vi "saveAllScanScripts.vi"(6 "scanType":string, 8 "error in (no error)":errorcluster, 9 "Values":string[](array[string]), 10 "scriptListArray":refnum<class "ScriptEventList.lvclass">[](array[class]), 11 "ScriptEditorV2 in":refnum<class "ScriptEditorV2.lvclass">) -> (0 "error out":errorcluster, 3 "ScriptEditorV2 out":refnum<class "ScriptEditorV2.lvclass">)   [LabVIEW 2009, in "Views.lvlib" / "ScriptEditor.lvlib" / "ScriptEditorV2.lvclass"]
uses:
  ScriptEditorV2.lvclass
  Tools/Scripting/ScriptingEvent/ScriptEventList/ScriptEventList.lvclass
  ScriptEditorV2.lvclass/ScriptEditorV2.ctl
  Tools/Scripting/DataPointScript/DataPointScript.lvclass
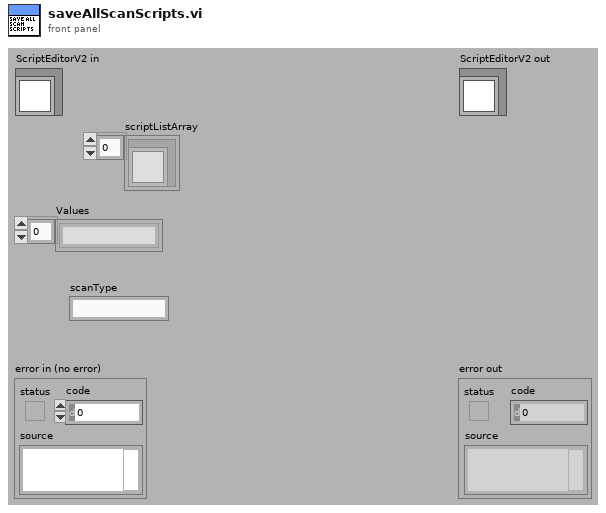
[diagram p1: front panel]
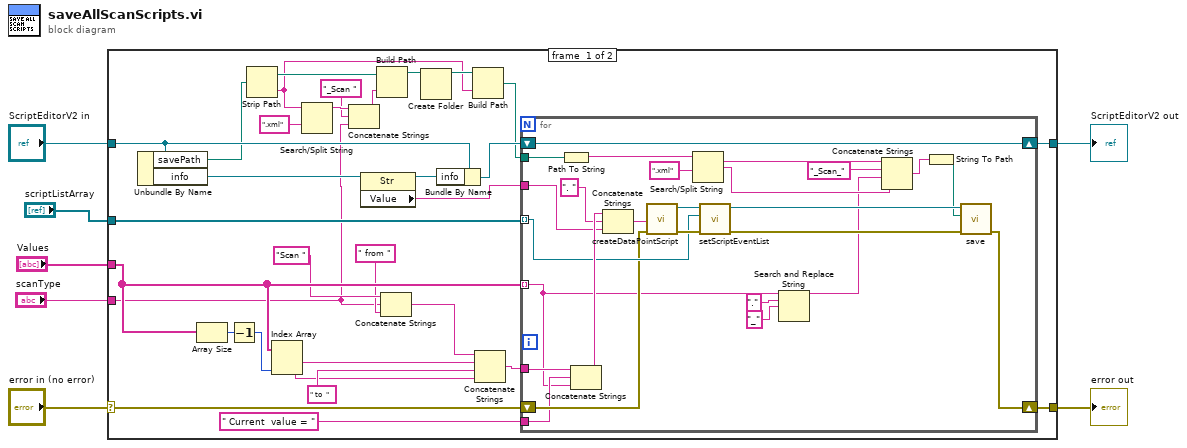
[diagram p0: block diagram]
diagram:
  n1 = case shown="No Error" "error in (no error)" {
    selector: "error in (no error)" -> [w37 w66]
    tunnel: [w38 w66] -> w6
    tunnel: [w36 w65] -> w4
    tunnel: "ScriptEditorV2 in" -> [w21 w65]
    tunnel: "scriptListArray" -> [w35 _]
    tunnel: "Values" -> [w34 _]
    tunnel: "scanType" -> [w8 _]
    frame #0 {
      n2 = Unbundle By Name(w21) -> ("savePath"=w18:path, "info"=w23:refnum<vi>)
      n3 = Array Size(array=w34) -> (size(s)=w33:i32)
      n4 = Decrement(x=w33) -> (x-1=w32:i32)
      n5 = Strip Path(path=w18) -> (stripped path=w17:path, name=w10:string)
      n6 = Index Array(array=w34, index #2=w32) -> (element #1=w31:string, element #2=w28:string)  [unwired: 1 in]
      n7 = Search/Split String(string=w10, search string/char (-)=".xml") -> (substring before match=w12:string)  [unwired: 1 in, 2 out]
      n8 = Concatenate Strings(w12, "_Scan ", w8) -> (w11:string)
      n9 = property class="Str"(reference=w23) -> (reference out=w19:refnum<vi>, "Value"=w22:string)  [unwired: 1 in, 1 out]
      n10 = Build Path(base path=w17, name or relative path=w11) -> (appended path=w16:path)
      n11 = Concatenate Strings("Scan ", w8, " from ") -> (w24:string)
      n12 = Create Folder(path (use dialog)=w16) -> (created path=w15:path)  [unwired: 2 in, 2 out]
      n13 = Bundle By Name(cluster=w21, "info"=w19) -> (w20:refnum<class "ScriptEditorV2.lvclass">)
      n14 = Build Path(base path=w15, name or relative path=w10) -> (appended path=w14:path)
      n15 = Concatenate Strings(w24, w31, " to  ", w28) -> (w27:string)
      n16 = for {
        shift-right: [w52] -> w38
        shift-left: w37 -> [w53]
        shift-right: [w64] -> w36
        shift-left: w20 -> [w64]
        tunnel: w35 -> [w54] mode=indexing
        tunnel: w34 -> [w39] mode=indexing
        tunnel: " Current  value = " -> [w40]
        tunnel: w27 -> [w63]
        tunnel: w22 -> [w56]
        tunnel: w14 -> [w51]
        n17 = Path To String(path=w51) -> (string=w47:string)
        n18 = Concatenate Strings(w63, w40, w39) -> (w57:string)
        n19 = Concatenate Strings(w57, ". ", w56) -> (w58:string)
        n20 = call "createDataPointScript.vi"("error in (no error)"=w53, "script_comment"=w58) -> ("error out"=w62:errorcluster, "DataPointScript out"=w61:refnum<class "DataPointScript.lvclass">)  [unwired: 8 in]
        n21 = Search/Split String(string=w47, search string/char (-)=".xml") -> (substring before match=w41:string, match + rest of string=w45:string)  [unwired: 1 in, 1 out]
        n22 = call "setScriptEventList.vi"("error in (no error)"=w62, "TScriptEventList"=w54, "DataPointScript.lvclass in"=w61) -> ("error out"=w60:errorcluster, "DataPointScript.lvclass out"=w59:refnum<class "DataPointScript.lvclass">)  [unwired: 7 in]
        n23 = Search and Replace String(input string=w39, search string=".", replace string="_") -> (result string=w42:string)  [unwired: 5 in, 3 out]
        n24 = Concatenate Strings(w41, "_Scan_", w42, w45) -> (w49:string)
        n25 = String To Path(string=w49) -> (path=w50:path)
        n26 = call "save.vi"("error in (no error)"=w60, "Path"=w50, "DataPointScript in"=w59) -> ("error out"=w52:errorcluster)  [unwired: 7 in, 1 out]
      }
    }
    frame #1 {
    }
  }
  "error out" <- w6
  "ScriptEditorV2 out" <- w4
